vi "WriteConfiguration_Decoration.vi"(7 "PythonConverter_GUI in":refnum<class "PythonConverter_GUI.lvclass">, 8 "error in":errorcluster, 11 "Decoration in":refnum<class "Decoration.lvclass">) -> (0 "error out":errorcluster, 3 "Decoration out":refnum<class "Decoration.lvclass">, 5 "PythonConverter_GUI out":refnum<class "PythonConverter_GUI.lvclass">)   [LabVIEW 2014, in "Raspberry Pi Compatible Compiler for LabVIEW.lvlib" / "PythonConverter_GUI.lvclass"]
uses:
  PythonConverter_GUI.lvclass
  VI Interpreter/Classes/Decoration/Decoration.lvclass
  PythonConverter_GUI.lvclass/PythonConverter_GUI.ctl
  PythonConfiguration/PythonConfiguration.lvclass/PythonConfiguration.ctl
  PythonConfiguration/PythonConfiguration.lvclass
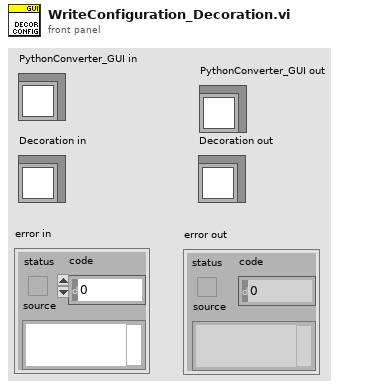
[diagram p1: front panel]
types:
  T1 = typedef "Raspberry Pi Compatible Compiler for LabVIEW.lvlib/PythonConfiguration.lvclass/ItemTD.ctl" = cluster{"Key":string, "Value":string}
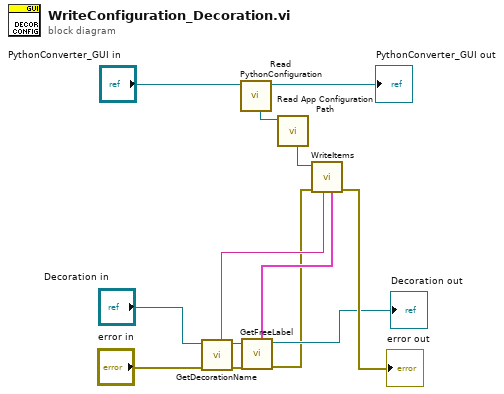
[diagram p0: block diagram]
diagram:
  n1 = call "GetDecorationName.vi"("error in"="error in", "Decoration in"="Decoration in") -> ("error out"=w3:errorcluster, "Decoration out"=w4:refnum<class "Decoration.lvclass">, "name"=w13:string)  [unwired: 5 in]
  n2 = call "Read PythonConfiguration.vi"("PythonConverter_GUI in"="PythonConverter_GUI in") -> ("PythonConverter_GUI out"=→"PythonConverter_GUI out":refnum<class "PythonConverter_GUI.lvclass">, "PythonConfiguration"=w10:refnum<class "PythonConfiguration.lvclass">)  [unwired: 7 in]
  n3 = call "GetFreeLabel.vi"("error in"=w3, "Decoration in"=w4) -> ("error out"=w1:errorcluster, "Decoration out"=→"Decoration out":refnum<class "Decoration.lvclass">, "Items"=w7:T1[])  [unwired: 5 in]
  n4 = call "Read App Configuration Path.vi"("PythonConfiguration in"=w10) -> ("App Configuration Path"=w9:path)  [unwired: 7 in, 1 out]
  n5 = call "WriteItems.vi"("Items"=w7, "section"=w13, "error in"=w1, "Path"=w9) -> ("error out"=→"error out":errorcluster)  [unwired: 5 in]
